vi "Sync to File.vi"(8 "error in (no error)":errorcluster, 9 "Write Reference?(F)":bool, 11 "CSM-Static-Variable-Manager in":refnum<class "CSM-Static-Variable-Manager.lvclass">) -> (0 "error out":errorcluster, 3 "CSM-Static-Variable-Manager out":refnum<class "CSM-Static-Variable-Manager.lvclass">)   [LabVIEW 2017, in "INI-Static-Variable-Support.lvlib" / "CSM-Static-Variable-Manager.lvclass"]
uses:
  CSM-Static-Variable-Manager.lvclass
  CSM-Static-Variable-Manager.lvclass/CSM-Static-Variable-Manager.ctl
  LabVIEW-Config/Config.ctl
  LabVIEW-Config/LineToken.ctl
  LabVIEW-Config/LabVIEW-Config.lvlib
  INI-Static-Variable-Support.lvlib
  <userlib>/_NEVSTOP/Communicable State Machine(CSM)/Communicable State Machine.lvlib
  <userlib>/_NEVSTOP/Communicable State Machine(CSM)/addons/API-String-Arugments-Support/API String Arguments Support.lvlib
  <userlib>/_NEVSTOP/Communicable State Machine(CSM)/_Shared/CSM Shared.lvlib
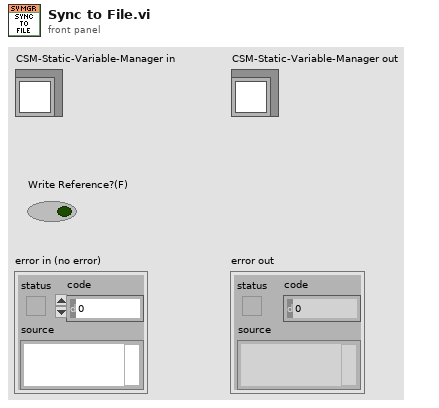
[diagram p1: front panel]
types:
  T1 = typedef "LabVIEW-Config.lvlib/Config.ctl" = cluster{"Path":path, "Lines":string[], "Tokens":T2[], "Modified?":bool}
  T2 = typedef "LabVIEW-Config.lvlib/LineToken.ctl" = enum8{"comment", "section", "key", "more"}
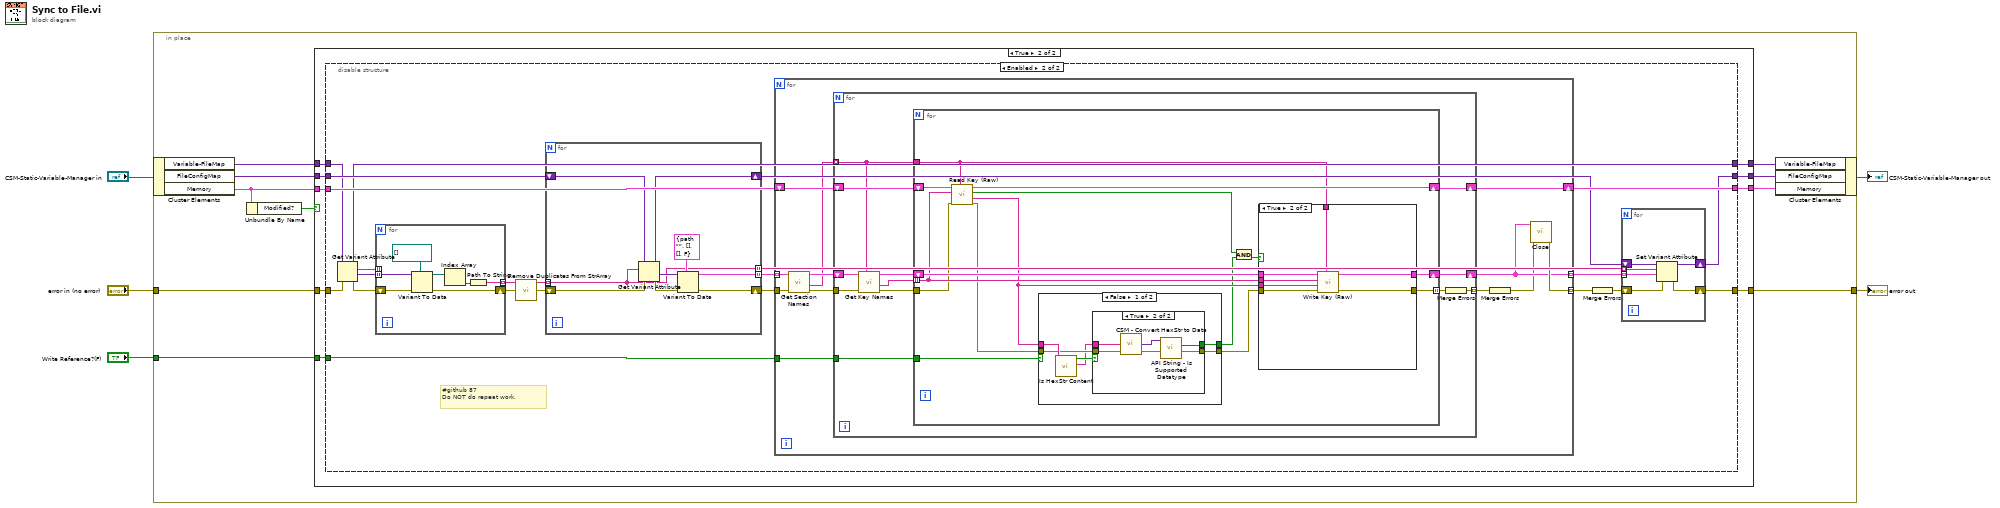
[diagram p0: block diagram]
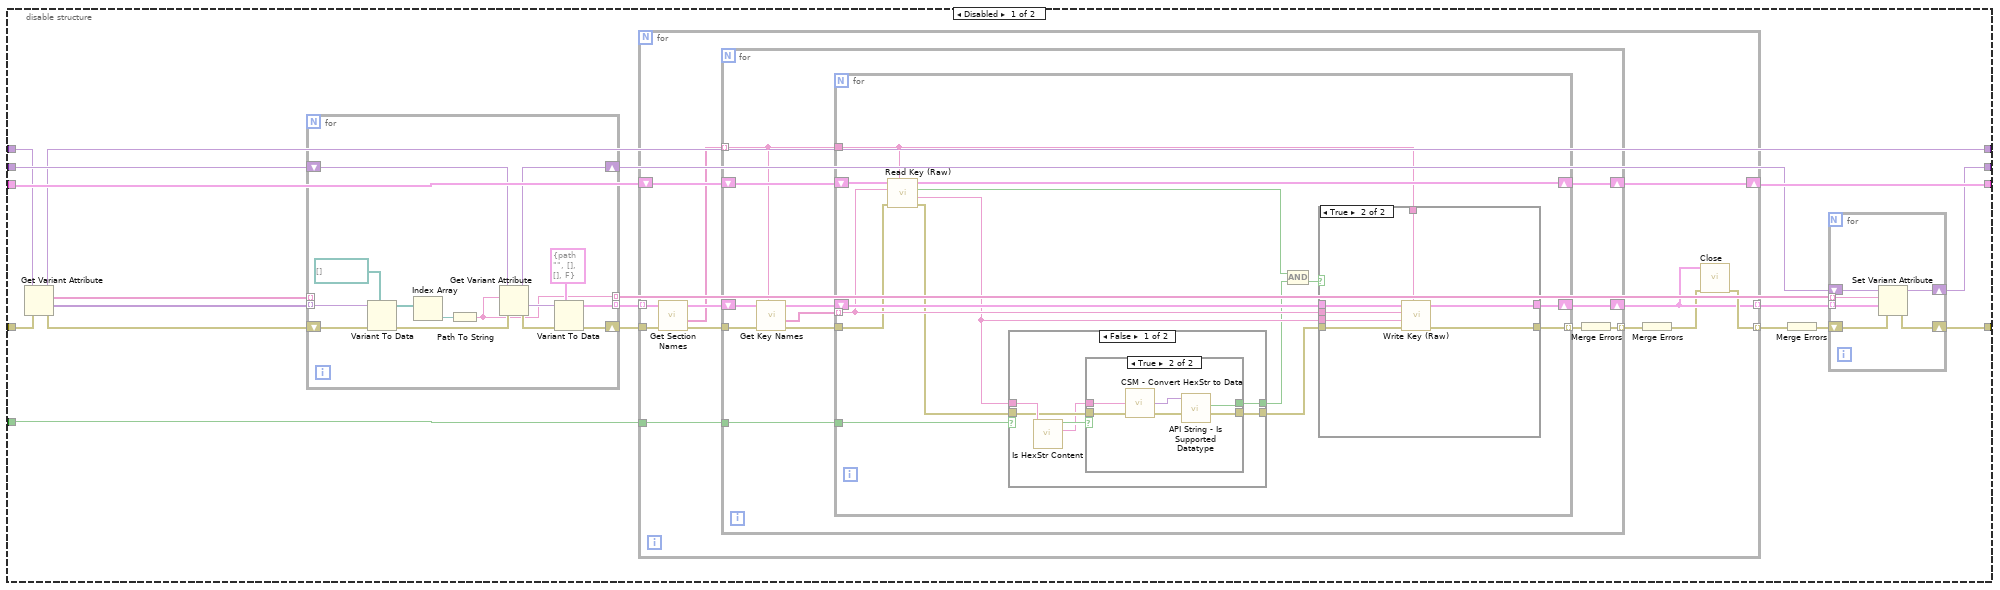
[diagram p3: hidden frame]
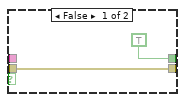
[diagram p4: hidden frame]
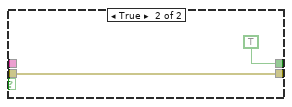
[diagram p5: hidden frame]
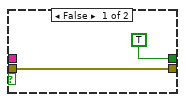
[diagram p7: hidden frame]
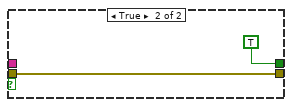
[diagram p8: hidden frame]
diagram:
  n1 = in-place {
    in-place-border: "error in (no error)" -> [w8]
    in-place-border: [w13] -> w2
    in-place-border: "Write Reference?(F)" -> [w11]
    n2 = in-place-cluster #1("CSM-Static-Variable-Manager in") -> ("Variable-FileMap"=w9:variant, "FileConfigMap"=w14:variant, "Memory"=w7:T1)
    n3 = Unbundle By Name(w7) -> ("Modified?"=w6:bool)
    n4 = case shown="True" w6 {
      tunnel: w7 -> [w17 w28]
      tunnel: [w17 w27] -> w15
      tunnel: w14 -> [w18 w26]
      tunnel: [w16 w25] -> w13
      tunnel: [w18 w24] -> w12
      tunnel: w11 -> [_ w23]
      tunnel: [w19 w22] -> w10
      tunnel: w9 -> [w19 w21]
      tunnel: w8 -> [w16 w20]
      frame False {
      }
      frame True {
        n5 = disable-structure shown="Enabled" {
          disable-tunnel: w28 -> [w47 w153]
          disable-tunnel: [w46 w152] -> w27
          disable-tunnel: w26 -> [w45 w151]
          disable-tunnel: [w42 w148] -> w25
          disable-tunnel: [w39 w145] -> w24
          disable-tunnel: w23 -> [w36 w142]
          disable-tunnel: [w34 w140] -> w22
          disable-tunnel: w21 -> [w33 w139]
          disable-tunnel: w20 -> [w30 w138]
          frame Disabled {
            n6 = Get Variant Attribute(Variant=w33, error in=w30) -> (duplicate Variant=w34:variant, names=w29:string[], values=w32:variant[], error out=w31:errorcluster)  [unwired: 2 in]
            n7 = for {
              tunnel: [w126] -> w43 mode=indexing
              tunnel: [w118] -> w37 mode=indexing
              tunnel: w32 -> [w123] mode=indexing
              shift-right: [w125] -> w40
              shift-left: w45 -> [w131]
              shift-right: [w128] -> w44
              shift-left: w31 -> [w122]
              tunnel: w29 -> [_] mode=indexing
              n8 = Variant To Data(error in=w122, type=path[] [], Variant=w123) -> (data=w120:path[], error out=w124:errorcluster)
              n9 = Index Array(array=w120) -> (element=w119:path)  [unwired: 1 in]
              n10 = Path To String(path=w119) -> (string=w118:string)
              n11 = Get Variant Attribute(Variant=w131, name=w118, error in=w124) -> (duplicate Variant=w125:variant, value=w130:variant, error out=w129:errorcluster)  [unwired: 1 in, 1 out]
              n12 = Variant To Data(error in=w129, type=T1 {"Path"=path "", "Lines"=[], "Tokens"=[], "Modified?"=FALSE}, Variant=w130) -> (data=w126:T1, error out=w128:errorcluster)
            }
            n13 = for {
              shift-right: [w63] -> w46
              shift-left: w47 -> [w64]
              tunnel: w43 -> [w65] mode=indexing
              tunnel: [w57] -> w38 mode=indexing
              tunnel: w36 -> [w55]
              tunnel: w44 -> [w61]
              tunnel: [w58] -> w41 mode=indexing
              n14 = call "Get Section Names.vi"("error in (no error)"=w61, "Config in"=w65) -> ("error out"=w60:errorcluster, "Section Names"=w59:string[], "Config out"=w62:T1)  [unwired: 7 in]
              n15 = for {
                shift-right: [w73] -> w63
                shift-left: w64 -> [w74]
                tunnel: w59 -> [w69] mode=indexing
                shift-right: [w68] -> w57
                shift-left: w62 -> [w71]
                tunnel: w55 -> [w67]
                tunnel: w60 -> [w70]
                tunnel: [w66] -> w56 mode=indexing
                n16 = call "Get Key Names.vi"("Section Name"=w69, "error in (no error)"=w70, "Config in"=w71) -> ("error out"=w75:errorcluster, "Key Names"=w76:string[], "Config out"=w77:T1)  [unwired: 5 in, 1 out]
                n17 = for {
                  tunnel: w69 -> [w89]
                  tunnel: w76 -> [w88] mode=indexing
                  shift-right: [w91] -> w73
                  shift-left: w74 -> [w90]
                  shift-right: [w85] -> w68
                  shift-left: w77 -> [w92]
                  tunnel: w67 -> [w80]
                  tunnel: w75 -> [w87]
                  tunnel: [w86] -> w72 mode=indexing
                  n18 = call "Read Key (Raw).vi"("Section Name"=w89, "error in (no error)"=w87, "Key Name"=w88, "Config in"=w90) -> ("error out"=w79:errorcluster, "Content"=w82:string, "Key Found?"=w83:bool, "Config out"=w91:T1)  [unwired: 4 in]
                  n19 = case shown="False" w80 {
                    tunnel: w82 -> [w98 _]
                    tunnel: [w94 TRUE ("HexStr Content")] -> w81
                    tunnel: w79 -> [w97 w107]
                    tunnel: [w96 w107] -> w78
                    frame False {
                      n20 = call "Is HexStr Content.vi"("Content"=w98) -> ("hexStr"=w93:string, "HexStr Content"=w95:bool)  [unwired: 9 in]
                      n21 = case shown="True" w95 {
                        tunnel: w93 -> [_ w106]
                        tunnel: w97 -> [w99 w105]
                        tunnel: [w99 w102] -> w96
                        tunnel: [TRUE ("HexStr Content") w101] -> w94
                        frame False {
                        }
                        frame True {
                          n22 = call <userlib>:"CSM - Convert HexStr to Data.vi"("HEX String"=w106, "error in (no error)"=w105) -> ("Variant"=w104:variant, "error out"=w103:errorcluster)  [unwired: 6 in]
                          n23 = call <userlib>:"API String - Is Supported Datatype.vi"("error in (no error)"=w103, "data"=w104) -> ("error out"=w102:errorcluster, "supported datatype?"=w101:bool)  [unwired: 7 in, 1 out]
                        }
                      }
                    }
                    frame True {
                    }
                  }
                  n24 = And(x=w83, y=w81) -> (x .and. y?=w84:bool)
                  n25 = case shown="True" w84 {
                    tunnel: w92 -> [w109 w117]
                    tunnel: w89 -> [_ w116]
                    tunnel: w88 -> [_ w115]
                    tunnel: [w110 w114] -> w86
                    tunnel: [w109 w113] -> w85
                    tunnel: w82 -> [_ w112]
                    tunnel: w78 -> [w110 w111]
                    frame False {
                    }
                    frame True {
                      n26 = call "Write Key (Raw).vi"("Section Name"=w116, "error in (no error)"=w111, "Content"=w112, "Key Name"=w115, "Config in"=w117) -> ("error out"=w114:errorcluster, "Config out"=w113:T1)  [unwired: 4 in, 1 out]
                    }
                  }
                }
                n27 = Merge Errors(w72) -> (w66:errorcluster)
              }
              n28 = Merge Errors(w56) -> (w54:errorcluster)
              n29 = call "Close.vi"("error in (no error)"=w54, "Config"=w57) -> ("error out"=w58:errorcluster)  [unwired: 8 in, 1 out]
            }
            n30 = Merge Errors(w41) -> (w35:errorcluster)
            n31 = for {
              shift-right: [w52] -> w42
              shift-left: w35 -> [w53]
              shift-right: [w50] -> w39
              shift-left: w40 -> [w51]
              tunnel: w38 -> [w49] mode=indexing
              tunnel: w37 -> [w48] mode=indexing
              n32 = Set Variant Attribute(Variant=w51, name=w48, value=w49, error in=w53) -> (Variant out=w50:variant, error out=w52:errorcluster)  [unwired: 1 out]
            }
          }
          frame Enabled {
            # "#github 87\nDo NOT do repeat work."
            n33 = Get Variant Attribute(Variant=w139, error in=w138) -> (duplicate Variant=w140:variant, names=w133:string[], values=w135:variant[], error out=w137:errorcluster)  [unwired: 2 in]
            n34 = for {
              tunnel: w135 -> [w166] mode=indexing
              shift-right: [w162] -> w136
              shift-left: w137 -> [w165]
              tunnel: [w160] -> w134 mode=indexing
              tunnel: w133 -> [_] mode=indexing
              n35 = Variant To Data(error in=w165, type=path[] [], Variant=w166) -> (data=w163:path[], error out=w162:errorcluster)
              n36 = Index Array(array=w163) -> (element=w161:path)  [unwired: 1 in]
              n37 = Path To String(path=w161) -> (string=w160:string)
            }
            n38 = call <userlib>:"Remove Duplicates From StrArray.vi"("StrArray in"=w134) -> ("StrArray"=w132:string[])  [unwired: 9 in, 1 out]
            n39 = for {
              tunnel: [w234] -> w149 mode=indexing
              tunnel: [w231] -> w143 mode=indexing
              shift-right: [w233] -> w146
              shift-left: w151 -> [w239]
              shift-right: [w236] -> w150
              shift-left: w136 -> [w232]
              tunnel: w132 -> [w231] mode=indexing
              n40 = Get Variant Attribute(Variant=w239, name=w231, error in=w232) -> (duplicate Variant=w233:variant, value=w238:variant, error out=w237:errorcluster)  [unwired: 1 in, 1 out]
              n41 = Variant To Data(error in=w237, type=T1 {"Path"=path "", "Lines"=[], "Tokens"=[], "Modified?"=FALSE}, Variant=w238) -> (data=w234:T1, error out=w236:errorcluster)
            }
            n42 = for {
              shift-right: [w176] -> w152
              shift-left: w153 -> [w177]
              tunnel: w149 -> [w178] mode=indexing
              tunnel: [w170] -> w144 mode=indexing
              tunnel: w142 -> [w168]
              tunnel: w150 -> [w174]
              tunnel: [w171] -> w147 mode=indexing
              n43 = call "Get Section Names.vi"("error in (no error)"=w174, "Config in"=w178) -> ("error out"=w173:errorcluster, "Section Names"=w172:string[], "Config out"=w175:T1)  [unwired: 7 in]
              n44 = for {
                shift-right: [w186] -> w176
                shift-left: w177 -> [w187]
                tunnel: w172 -> [w182] mode=indexing
                shift-right: [w181] -> w170
                shift-left: w175 -> [w184]
                tunnel: w168 -> [w180]
                tunnel: w173 -> [w183]
                tunnel: [w179] -> w169 mode=indexing
                n45 = call "Get Key Names.vi"("Section Name"=w182, "error in (no error)"=w183, "Config in"=w184) -> ("error out"=w188:errorcluster, "Key Names"=w189:string[], "Config out"=w190:T1)  [unwired: 5 in, 1 out]
                n46 = for {
                  tunnel: w182 -> [w202]
                  tunnel: w189 -> [w201] mode=indexing
                  shift-right: [w204] -> w186
                  shift-left: w187 -> [w203]
                  shift-right: [w198] -> w181
                  shift-left: w190 -> [w205]
                  tunnel: w180 -> [w193]
                  tunnel: w188 -> [w200]
                  tunnel: [w199] -> w185 mode=indexing
                  n47 = call "Read Key (Raw).vi"("Section Name"=w202, "error in (no error)"=w200, "Key Name"=w201, "Config in"=w203) -> ("error out"=w192:errorcluster, "Content"=w195:string, "Key Found?"=w196:bool, "Config out"=w204:T1)  [unwired: 4 in]
                  n48 = case shown="False" w193 {
                    tunnel: w195 -> [w211 _]
                    tunnel: [w207 TRUE ("HexStr Content")] -> w194
                    tunnel: w192 -> [w210 w220]
                    tunnel: [w209 w220] -> w191
                    frame False {
                      n49 = call "Is HexStr Content.vi"("Content"=w211) -> ("hexStr"=w206:string, "HexStr Content"=w208:bool)  [unwired: 9 in]
                      n50 = case shown="True" w208 {
                        tunnel: w206 -> [_ w219]
                        tunnel: w210 -> [w212 w218]
                        tunnel: [w212 w215] -> w209
                        tunnel: [TRUE ("HexStr Content") w214] -> w207
                        frame False {
                        }
                        frame True {
                          n51 = call <userlib>:"CSM - Convert HexStr to Data.vi"("HEX String"=w219, "error in (no error)"=w218) -> ("Variant"=w217:variant, "error out"=w216:errorcluster)  [unwired: 6 in]
                          n52 = call <userlib>:"API String - Is Supported Datatype.vi"("error in (no error)"=w216, "data"=w217) -> ("error out"=w215:errorcluster, "supported datatype?"=w214:bool)  [unwired: 7 in, 1 out]
                        }
                      }
                    }
                    frame True {
                    }
                  }
                  n53 = And(x=w196, y=w194) -> (x .and. y?=w197:bool)
                  n54 = case shown="True" w197 {
                    tunnel: w205 -> [w222 w230]
                    tunnel: w202 -> [_ w229]
                    tunnel: w201 -> [_ w228]
                    tunnel: [w223 w227] -> w199
                    tunnel: [w222 w226] -> w198
                    tunnel: w195 -> [_ w225]
                    tunnel: w191 -> [w223 w224]
                    frame False {
                    }
                    frame True {
                      n55 = call "Write Key (Raw).vi"("Section Name"=w229, "error in (no error)"=w224, "Content"=w225, "Key Name"=w228, "Config in"=w230) -> ("error out"=w227:errorcluster, "Config out"=w226:T1)  [unwired: 4 in, 1 out]
                    }
                  }
                }
                n56 = Merge Errors(w185) -> (w179:errorcluster)
              }
              n57 = Merge Errors(w169) -> (w167:errorcluster)
              n58 = call "Close.vi"("error in (no error)"=w167, "Config"=w170) -> ("error out"=w171:errorcluster)  [unwired: 8 in, 1 out]
            }
            n59 = Merge Errors(w147) -> (w141:errorcluster)
            n60 = for {
              shift-right: [w158] -> w148
              shift-left: w141 -> [w159]
              shift-right: [w156] -> w145
              shift-left: w146 -> [w157]
              tunnel: w144 -> [w155] mode=indexing
              tunnel: w143 -> [w154] mode=indexing
              n61 = Set Variant Attribute(Variant=w157, name=w154, value=w155, error in=w159) -> (Variant out=w156:variant, error out=w158:errorcluster)  [unwired: 1 out]
            }
          }
        }
      }
    }
    n62 = in-place-cluster #1("Variable-FileMap"=w10, "FileConfigMap"=w12, "Memory"=w15) -> (→"CSM-Static-Variable-Manager out":refnum<class "CSM-Static-Variable-Manager.lvclass">)
  }
  "error out" <- w2
